vi "Analysis-Redirector.vi"(8 "error in (no error)":errorcluster, 9 "VI reference":refnum<vi>, 11 "selected path":path) -> (0 "error out":errorcluster, 1 "PTP (Out)":dbl, 2 "SGP":dbl, 3 "error?":bool, 5 "Interruption Time (Out)":dbl)   [LabVIEW 2013]
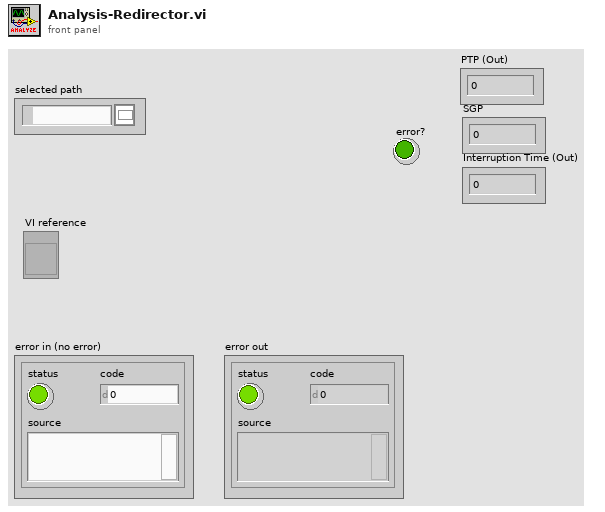
[diagram p1: front panel]
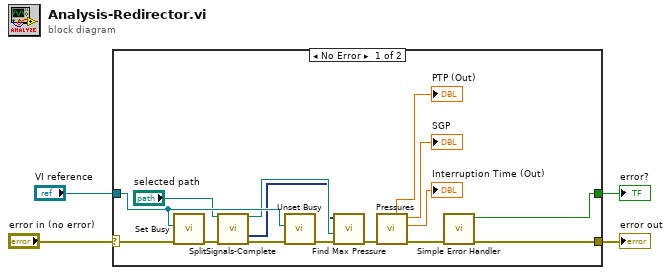
[diagram p0: block diagram]
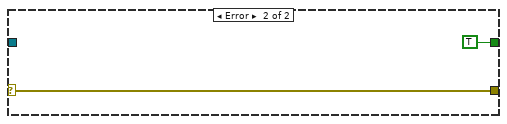
[diagram p2: hidden frame]
diagram:
  n1 = case shown="No Error" "error in (no error)" {
    selector: "error in (no error)" -> [w19 w21]
    tunnel: [w16 w21] -> w4
    tunnel: "VI reference" -> [w18 _]
    tunnel: [w15 TRUE ("error?")] -> w1
    frame No Error {
      n2 = call <vilib>:"Set Busy.vi"("error in (no error)"=w19, "VI reference (current VI)"=w18) -> ("error out"=w10:errorcluster)  [unwired: 8 in, 1 out]
      n3 = call "SplitSignals-Complete.vi"("Filename"="selected path", "Error In"=w10) -> ("Filename Out"=w6:path, "Pressure"=w5:dynamicdata, "Error Out"=w11:errorcluster)  [unwired: 10 in, 1 out]
      n4 = call <vilib>:"Unset Busy.vi"("error in (no error)"=w11, "VI reference (current VI)"=w18) -> ("error out"=w7:errorcluster)  [unwired: 9 in]
      n5 = call "Find Max Pressure.vi"("Error In"=w7, "File Path"=w6, "Pressure"=w5) -> ("Error Out"=w8:errorcluster)  [unwired: 4 in, 3 out]
      n6 = call "Pressures.vi"("Error In"=w8) -> ("Error Out"=w17:errorcluster, "Interruption Time"=→"Interruption Time (Out)":dbl, "SGP"=→"SGP":dbl, "PTP"=→"PTP (Out)":dbl)  [unwired: 6 in, 1 out]
      n7 = call <vilib>:"Simple Error Handler.vi"("error in (no error)"=w17) -> ("error?"=w15:bool, "error out"=w16:errorcluster)  [unwired: 4 in, 3 out]
    }
    frame Error {
    }
  }
  "error out" <- w4
  "error?" <- w1
